vi "Table Set Cell Size.vi"(9 "Cell Size":T1={"Width"=27, "Height"=20}, 10 "Cells":cluster{"Row":i32, "Column":i32}={"Row"=100, "Column"=100}, 11 "Table Ref In":refnum<vi>) -> (3 "Table Ref Out":refnum<vi>)   [LabVIEW 2024]
uses:
  <vilib>/Utility/miscctls.llb/LVBoundsTypeDef.ctl
  <vilib>/Utility/miscctls.llb/LVRowAndColumnTypeDef.ctl
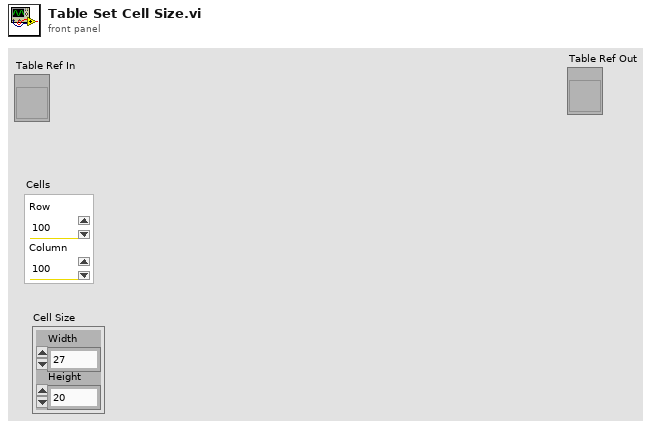
[diagram p1: front panel]
types:
  T1 = typedef "LVBoundsTypeDef.ctl" = cluster{"Width":u32, "Height":u32}
  T2 = typedef "LVRowAndColumnTypeDef.ctl" = cluster{"Row":i32, "Column":i32}
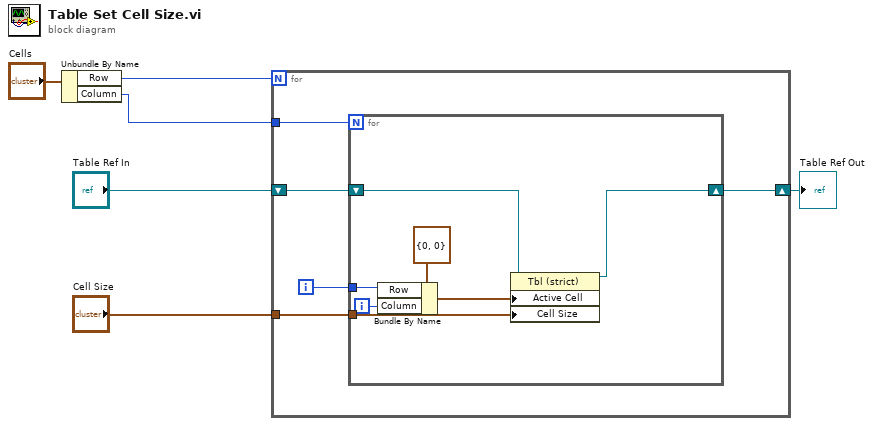
[diagram p0: block diagram]
diagram:
  n1 = Unbundle By Name("Cells") -> ("Row"=w2:i32, "Column"=w1:i32)
  n2 = for {
    N: w2 -> [_]
    tunnel: w1 -> [w10]
    shift-right: [w8] -> w5
    shift-left: "Table Ref In" -> [w9]
    tunnel: "Cell Size" -> [w7]
    i -> [w11]
    n3 = for {
      N: w10 -> [_]
      tunnel: w11 -> [w17]
      shift-right: [w13] -> w8
      shift-left: w9 -> [w14]
      tunnel: w7 -> [w12]
      i -> [w16]
      n4 = Bundle By Name(cluster=T2 {"Row"=0, "Column"=0} ("Active Cell:Active Cell"), "Row"=w17, "Column"=w16) -> (w15:T2)
      n5 = property on="Property Node" class="Tbl (strict)"(reference=w14, "Active Cell"=w15, "Cell Size"=w12) -> (reference out=w13:refnum<vi>)  [unwired: 1 in, 1 out]
    }
  }
  "Table Ref Out" <- w5
